vi "Set Telemetry Parameters.vi"(10 "MICS_Config_In":T1={"ConfigFlags"=0, "ImplantID"=1048576, "CompanyID"=187, "Normal_Comm"={"RF_Channel"=2, "UserData"=0, "TX_Mod"=0, "RX_Mod"=0, "RX_BlockSize"=15, "BlockPerPack"=31, "TX_BlockSize"=15}, "Emerg_Comm"={"RF_Channel"=2, "UserData"=0, "TX_Mod"=0, "RX_Mod"=0, "TX_BlockSize"=15, "BlockPerPack"=31, "RX_BlockSize"=15}, "ImplantRev"=4, "245TX_PowerCal"=0, "245TX_Power"=6, "CCA_RSSI_Thresholds"={"ch0"=2650, "ch1"=2650, "ch2"=2650, "ch3"=2650, "ch4"=2650, "ch5"=2650, "ch6"=2650, "ch7"=2650, "ch8"=2650, "ch9"=2650}} {"Normal_Comm"."RF_Channel" items=["0", "1", "2", "3", "4", "5", "6", "7", "8", "9"]; "Normal_Comm"."UserData" items=["0 - 000"=0, "1 - 001"=16, "2 - 010"=32, "3 - 011"=48, "4 - 100"=64, "5 - 101"=80, "6 - 110"=96, "7 - 111"=112]; "Normal_Comm"."TX_Mod" items=["2FSK-FB"=0, "2FSK"=2, "4FSK"=3]; "Normal_Comm"."RX_Mod" items=["2FSK-FB"=0, "2FSK"=8, "4FSK"=12]; "Normal_Comm"."RX_BlockSize" items=["2"=2, "3"=3, "4"=4, "5"=5, "6"=6, "7"=7, "8"=8, "9"=9, "10"=10, "11"=11, "12"=12, "13"=13, "14"=14, "15"=15, "16"=16, "17"=17, "18"=18, "19"=19, "20"=20, "21"=21, "22"=22, "23"=23, "24"=24, "25"=25, "26"=26, "27"=27, "28"=28, "29"=29, "30"=30, "31"=31]; "Normal_Comm"."BlockPerPack" items=["1"=1, "2"=2, "3"=3, "4"=4, "5"=5, "6"=6, "7"=7, "8"=8, "9"=9, "10"=10, "11"=11, "12"=12, "13"=13, "14"=14, "15"=15, "16"=16, "17"=17, "18"=18, "19"=19, "20"=20, "21"=21, "22"=22, "23"=23, "24"=24, "25"=25, "26"=26, "27"=27, "28"=28, "29"=29, "30"=30, "31"=31]; "Normal_Comm"."TX_BlockSize" items=["2"=2, "3"=3, "4"=4, "5"=5, "6"=6, "7"=7, "8"=8, "9"=9, "10"=10, "11"=11, "12"=12, "13"=13, "14"=14, "15"=15, "16"=16, "17"=17, "18"=18, "19"=19, "20"=20, "21"=21, "22"=22, "23"=23, "24"=24, "25"=25, "26"=26, "27"=27, "28"=28, "29"=29, "30"=30, "31"=31]; "Emerg_Comm"."RF_Channel" items=["0", "1", "2", "3", "4", "5", "6", "7", "8", "9"]; "Emerg_Comm"."UserData" items=["0 - 000"=0, "1 - 001"=16, "2 - 010"=32, "3 - 011"=48, "4 - 100"=64, "5 - 101"=80, "6 - 110"=96, "7 - 111"=112]; "Emerg_Comm"."TX_Mod" items=["2FSK-FB"=0, "2FSK"=2, "4FSK"=3]; "Emerg_Comm"."RX_Mod" items=["2FSK-FB"=0, "2FSK"=8, "4FSK"=12]; "Emerg_Comm"."TX_BlockSize" items=["2"=2, "3"=3, "4"=4, "5"=5, "6"=6, "7"=7, "8"=8, "9"=9, "10"=10, "11"=11, "12"=12, "13"=13, "14"=14, "15"=15, "16"=16, "17"=17, "18"=18, "19"=19, "20"=20, "21"=21, "22"=22, "23"=23, "24"=24, "25"=25, "26"=26, "27"=27, "28"=28, "29"=29, "30"=30, "31"=31]; "Emerg_Comm"."BlockPerPack" items=["1"=1, "2"=2, "3"=3, "4"=4, "5"=5, "6"=6, "7"=7, "8"=8, "9"=9, "10"=10, "11"=11, "12"=12, "13"=13, "14"=14, "15"=15, "16"=16, "17"=17, "18"=18, "19"=19, "20"=20, "21"=21, "22"=22, "23"=23, "24"=24, "25"=25, "26"=26, "27"=27, "28"=28, "29"=29, "30"=30, "31"=31]; "Emerg_Comm"."RX_BlockSize" items=["2"=2, "3"=3, "4"=4, "5"=5, "6"=6, "7"=7, "8"=8, "9"=9, "10"=10, "11"=11, "12"=12, "13"=13, "14"=14, "15"=15, "16"=16, "17"=17, "18"=18, "19"=19, "20"=20, "21"=21, "22"=22, "23"=23, "24"=24, "25"=25, "26"=26, "27"=27, "28"=28, "29"=29, "30"=30, "31"=31]; "ImplantRev" items=["ZL70100"=0, "ZL70101"=1, "ZL70102"=4]; "245TX_PowerCal" items=["-29"=-29, "-4"=-4, "-2"=-2, "0"=0, "2"=2, "4"=4, "6"=6, "8"=8, "10"=10, "12"=12, "14"=14, "16"=16, "18"=18, "20"=20, "22"=22, "24"=24, "26"=26, "27"=27]; "245TX_Power" items=["-29"=-29, "-4"=-4, "-2"=-2, "0"=0, "2"=2, "4"=4, "6"=6, "8"=8, "10"=10, "12"=12, "14"=14, "16"=16, "18"=18, "20"=20, "22"=22, "24"=24, "26"=26, "27"=27]}) -> ()   [LabVIEW 2020]
uses:
  MICS Parameters Global.vi
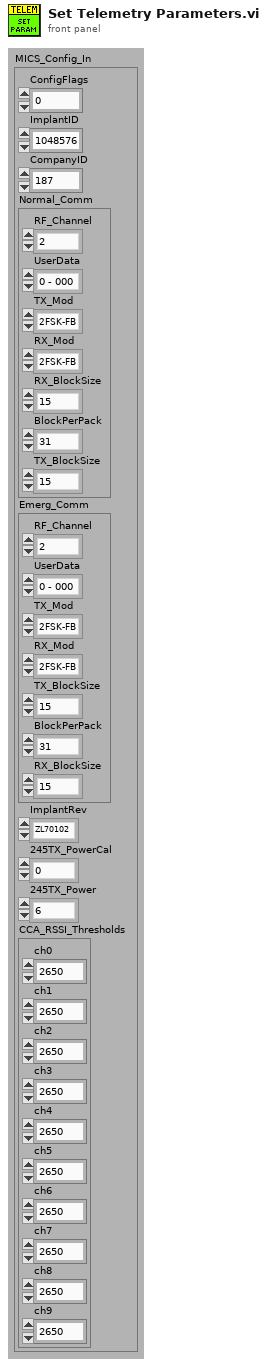
[diagram p1: front panel]
types:
  T1 = cluster{"ConfigFlags":u8, "ImplantID":u32, "CompanyID":u8, "Normal_Comm":cluster{"RF_Channel":u8, "UserData":u8, "TX_Mod":u8, "RX_Mod":u8, "RX_BlockSize":u8, "BlockPerPack":u8, "TX_BlockSize":u8}, "Emerg_Comm":cluster{"RF_Channel":u8, "UserData":u8, "TX_Mod":u8, "RX_Mod":u8, "TX_BlockSize":u8, "BlockPerPack":u8, "RX_BlockSize":u8}, "ImplantRev":u8, "245TX_PowerCal":i8, "245TX_Power":i8, "CCA_RSSI_Thresholds":cluster{"ch0":u16, "ch1":u16, "ch2":u16, "ch3":u16, "ch4":u16, "ch5":u16, "ch6":u16, "ch7":u16, "ch8":u16, "ch9":u16}}
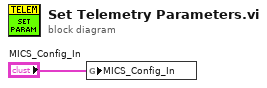
[diagram p0: block diagram]
diagram:
  n1 = global write "MICS Parameters Global.vi" "MICS_Config_In"("MICS_Config_In") -> ()
